vi "http upgrade action.vi"(9 "plugins":T1, 10 "tcp conn":refnum<k5>, 11 "application request in":T2) -> ()   [LabVIEW 2013]
uses:
  http request.ctl
  http method.ctl
  http plugins.ctl
  http upgrade callback.ctl
  http upgrade data.ctl
panel:
  out "error IO":errorcluster
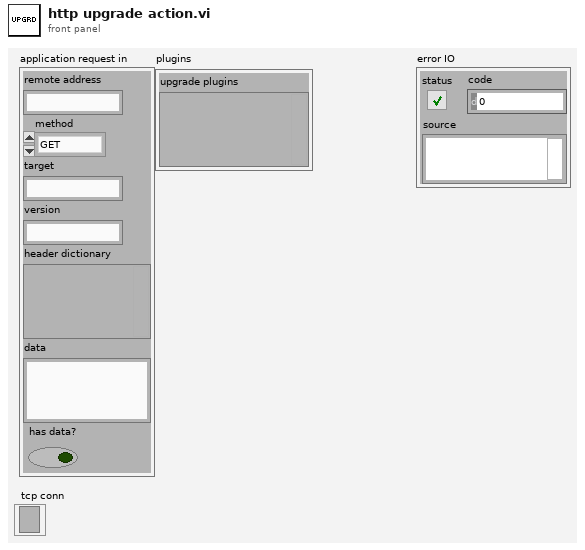
[diagram p1: front panel]
types:
  T1 = typedef "http plugins.ctl" = cluster{"upgrade plugins":variant}
  T2 = typedef "http request.ctl" = cluster{"remote address":string, "method":T3, "target":string, "version":string, "header dictionary":variant, "data":string, "has data?":bool}
  T3 = typedef "http method.ctl" = enum16{"GET", "POST", "PUT", "DELETE", "HEAD", "OPTIONS", "upgrade"}
  T4 = typedef "http upgrade callback.ctl" = cluster{"callback":refnum<vi>, "parameters":variant}
  T5 = typedef "http upgrade data.ctl" = cluster{"TCP connection":refnum<k5>, "application request":T2}
  T6 = typedef "http response.ctl" = cluster{"packet type":T7, "version":string, "reason code":u16, "status string":string, "header dictionary":variant, "cookies":string[], "data":string}
  T7 = typedef "http response packet type.ctl" = enum16{"full response", "header only", "data only", "last data"}
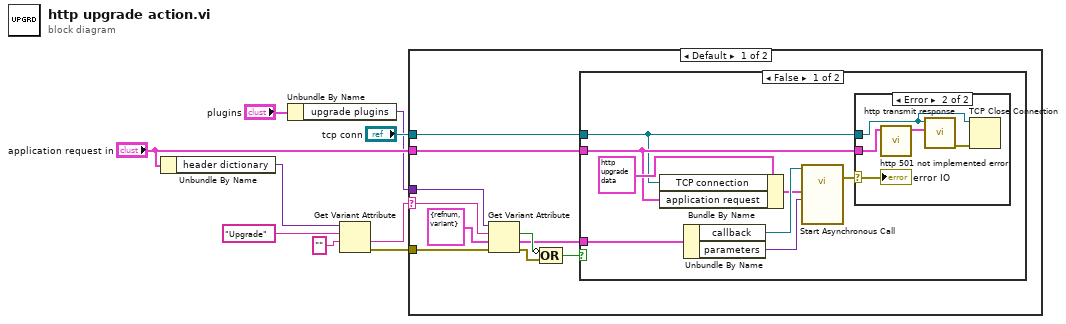
[diagram p0: block diagram]
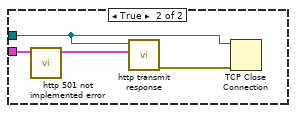
[diagram p3: hidden frame]
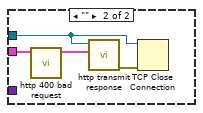
[diagram p4: hidden frame]
diagram:
  n1 = Unbundle By Name("application request in") -> ("header dictionary"=w9:variant)
  n2 = Unbundle By Name("plugins") -> ("upgrade plugins"=w2:variant)
  n3 = Get Variant Attribute(Variant=w9, name="Upgrade", default value (empty Variant)="" ("name")) -> (value=w6:string, error out=w1:errorcluster)  [unwired: 1 in, 2 out]
  n4 = case shown="Default" w6 {
    selector: w6 -> [w14 _]
    tunnel: "tcp conn" -> [w19 w39]
    tunnel: "application request in" -> [w18 w37]
    tunnel: w2 -> [w17 _]
    tunnel: w1 -> [w16 _]
    frame Default {
      n5 = Get Variant Attribute(Variant=w17, name=w14, default value (empty Variant)=T4 {"callback"=refnum, "parameters"=variant} ("callback"), error in=w16) -> (found=w13:bool, value=w10:T4, error out=w12:errorcluster)  [unwired: 1 out]
      n6 = Compound Arithmetic op=OR(invert w13, w12) -> (w11:bool)
      n7 = case shown="False" w11 {
        tunnel: w19 -> [w20 w35]
        tunnel: w18 -> [w21 w33]
        tunnel: w10 -> [w27 _]
        frame False {
          n8 = Bundle By Name(cluster=T5 {"TCP connection"=refnum, "application request"={"remote address"="", "method"=enum."GET", "target"="", "version"="", "header dictionary"=variant, "data"="", "has data?"=FALSE}} ("upgrade data"), "TCP connection"=w20, "application request"=w21) -> (w23:T5)
          n9 = Unbundle By Name(w27) -> ("callback"=w26:refnum<vi>, "parameters"=w25:variant)
          n10 = call-by-ref "Start Asynchronous Call"(reference=w26, "parameters"=w25, "upgrade data"=w23) -> (error out=w22:errorcluster)  [unwired: 11 in, 1 out]
          n11 = case shown="Error" w22 {
            selector: w22 -> [_ w28]
            tunnel: w21 -> [_ w30]
            tunnel: w20 -> [_ w29]
            frame No Error {
            }
            frame Error {
              n12 = call "http 501 not implemented error.vi"("application request in"=w30) -> ("application request out"=w31:T6)  [unwired: 10 in]
              n13 = call "http transmit response.vi"("application request"=w31, "tcp connection"=w29) -> ("error out"=w32:errorcluster)  [unwired: 9 in]
              n14 = TCP Close Connection(connection ID=w29, error in (no error)=w32) -> ()  [unwired: 1 in, 2 out]
              "error IO" <- w28
            }
          }
        }
        frame True {
          n15 = call "http 501 not implemented error.vi"("application request in"=w33) -> ("application request out"=w34:T6)  [unwired: 10 in]
          n16 = call "http transmit response.vi"("application request"=w34, "tcp connection"=w35) -> ("error out"=w36:errorcluster)  [unwired: 9 in]
          n17 = TCP Close Connection(connection ID=w35, error in (no error)=w36) -> ()  [unwired: 1 in, 2 out]
        }
      }
    }
    frame "" {
      n18 = call "http 400 bad request.vi"("application request in"=w37) -> ("application request out"=w38:T6)  [unwired: 10 in]
      n19 = call "http transmit response.vi"("application request"=w38, "tcp connection"=w39) -> ("error out"=w40:errorcluster)  [unwired: 9 in]
      n20 = TCP Close Connection(connection ID=w39, error in (no error)=w40) -> ()  [unwired: 1 in, 2 out]
    }
  }
